vi "Init UART.vi"(4 "TX GPIO":T1=16, 5 "Term Char (None)":string, 6 "RX GPIO":T1=17, 7 "UART #":T2, 8 "error in (no error)":errorcluster, 10 "Baud":u32=115200, 11 "VisaSession in":refnum<class "VisaSession.lvclass">) -> (0 "error out":errorcluster, 2 "UART":refnum<class "UART.lvclass">, 3 "VisaSession out":refnum<class "VisaSession.lvclass">)   [LabVIEW 2020, in "CTI.lvlib" / "VisaSession.lvclass"]
uses:
  VisaSession.lvclass
  VisaSession.lvclass/VisaSession.ctl
  Session/Session.lvclass
  UART Number.ctl
  CTI.lvlib
  GPIO Number.ctl
  UART/UART.lvclass
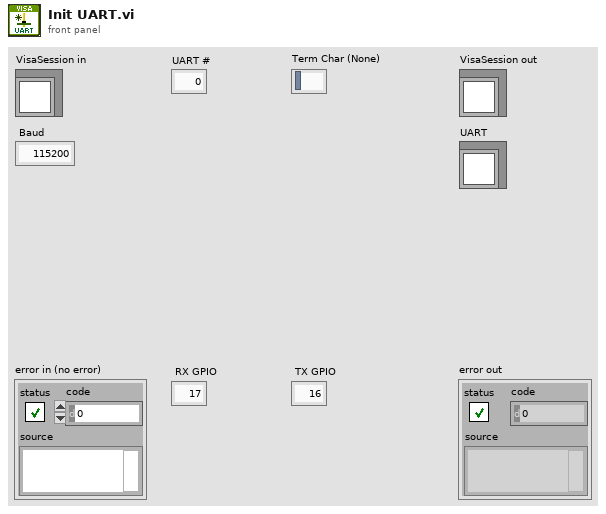
[diagram p1: front panel]
types:
  T1 = typedef "CTI.lvlib/GPIO Number.ctl" = i8
  T2 = typedef "CTI.lvlib/UART Number.ctl" = i8
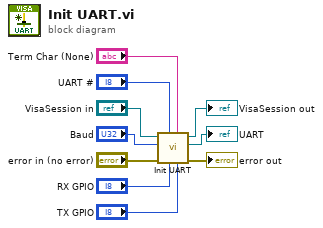
[diagram p0: block diagram]
diagram:
  n1 = call-parent "Init UART.vi"("TX GPIO"="TX GPIO", "Term Char (None)"="Term Char (None)", "RX GPIO"="RX GPIO", "UART #"="UART #", "error in (no error)"="error in (no error)", "Baud"="Baud", "Session in"="VisaSession in") -> ("error out"=→"error out":errorcluster, "UART"=→"UART":refnum<class "UART.lvclass">, "Session out"=→"VisaSession out":refnum<class "VisaSession.lvclass">)  [unwired: 2 in]
